vi "Get Request Type.vi"(8 "error in (no error)":errorcluster, 11 "GetSourceScreenshot in":refnum<class "GetSourceScreenshot.lvclass">) -> (0 "error out":errorcluster, 2 "Request Type":string, 3 "GetSourceScreenshot out":refnum<class "GetSourceScreenshot.lvclass">)   [LabVIEW 2020, in "obs-websocket.lvlib" / "GetSourceScreenshot.lvclass"]
uses:
  GetSourceScreenshot.lvclass
  GetSourceScreenshot.lvclass/GetSourceScreenshot.ctl
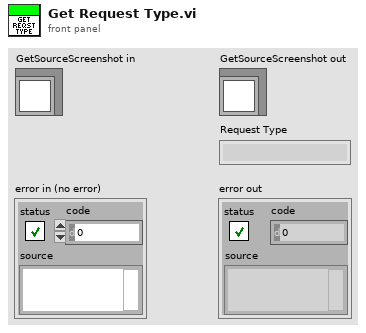
[diagram p1: front panel]
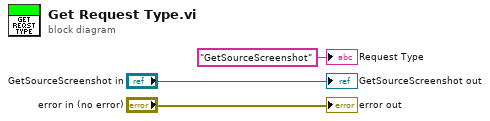
[diagram p0: block diagram]
diagram:
  "error out" <- "error in (no error)"
  "GetSourceScreenshot out" <- "GetSourceScreenshot in"
  "Request Type" <- "GetSourceScreenshot" ("Request Type")
